vi "Confocal_0919.vi"() -> ()   [LabVIEW 2017]
uses:
  <vilib>/Math Plots/2D Math Plots/XY Plot Matrix/XY Plot Matrix XCtrl/XY Plot Matrix.xctl
  Public/Documents/SIToolkit/LabVIEW/ExamplesXX_4_3_1_4/Spectroscopy Applications/GlobalCamOpen.vi
  Public/Documents/SIToolkit/LabVIEW/ExamplesXX_4_3_1_4/Spectroscopy Applications/GlobalInitializeFlag.vi
  Program Files/SITK/SIToolkit/LabVIEW/ExamplesXX_4_3_1_4/Adv Applications/GlobalTimingMode.vi
  Public/Documents/SIToolkit/LabVIEW/ExamplesXX_4_3_1_4/Spectroscopy Applications/GlobalFramesToStr.vi
  Public/Documents/SIToolkit/LabVIEW/ExamplesXX_4_3_1_4/Spectroscopy Applications/GlobalAcquireFocusFlag.vi
  Public/Documents/SIToolkit/LabVIEW/ExamplesXX_4_3_1_4/Spectroscopy Applications/GlobalExposure.vi
  <vilib>/Math Plots/2D Math Plots/XY Plot Matrix/XY Plot Matrix Datatype/XY Plot Matrix Datatype.lvclass
panel:
  out "Position 7":dbl[](array[numeric]) format="%.6f"
  out "Position 4":dbl[](array[numeric]) format="%.6f"
  in  "error PI Stage":errorcluster
  out "error out 2":errorcluster
  in  "Tab Control":T1(tab)
  in  "Focus/Acquire Mode":u32=1 min=1 max=5 step=1
  in  "Number of Frames to store":u32=1 min=1 step=1
  in  "Timing Mode":u32(ring)=1 items=["N/A", "Free Run/Timed", "Trigger First (PM only)", "Ext Sync/Strobed ", "Variable Exp (PM only)", "Flash Mode (PM only)"]
  out "Pixel Time":i32
  out "Bit Depth":i32
  out "ReadOut port":i32
  out "ADC Speed":i32
  in  "Set Experiment \nParameters, Initialize \nCamera/Controller":bool
  out "Read Temp.":dbl format="%.2f"
  in  "Set Temp.":dbl format="%.2f"
  in  "Exposure 2":dbl=0.2 format="%.2f"
  out "Controller Initialized":bool
  in  "error in":errorcluster
  out "error out":errorcluster
  in  "Power":dbl=10.0
  in  "RF Power":bool=TRUE
  in  "Frequency":dbl=2810.0
  in  "Release Camera":bool
  out "Position 6":dbl[](array[numeric]) format="%.6f"
  out "Conn. Axis 5":string[](array[string])
  out "error out 3":errorcluster
  in  "stop":bool
  out "Read Frequency":dbl
  in  "Initial Frequency":dbl=2820.0
  in  "Final Frequency":dbl=2890.0
  in  "Step Size":dbl=3.0
  in  "OK Button 3":bool
  out "XY Plot Matrix":refnum<class "XY Plot Matrix Datatype.lvclass">[](xcontrol)
  out "history":dbl[][](array[numeric])
  in  "Number of Scans":i32
  in  "Serial Port":refnum<visa-resource-name>="COM3"
  out "COM Error":bool
  out "Camera Opened":bool
  out "Scan":i32
  in  "Number of Steps Left":dbl=5.0 format="%#_13g"
  in  "OK Button 5":bool
  in  "Step Size (microns)":dbl[](array[numeric])=[0.01]
  out "XY Plot Matrix":refnum<class "XY Plot Matrix Datatype.lvclass">[](xcontrol)
  in  "Number of Steps Down":dbl=5.0 format="%#_13g"
  out "Position":dbl[](array[numeric]) format="%.6f"
  out "Position 3":dbl[](array[numeric]) format="%.6f"
  in  "stop 2":bool
  out "Line Number":i32
  out "Position 2":dbl[](array[numeric]) format="%.6f"
  in  "?":bool
  out "Position 5":dbl[](array[numeric]) format="%.6f"
  in  "Step Size (microns) Y":dbl[](array[numeric])=[0.01]
  in  "Step Size (microns) X":dbl[](array[numeric])=[0.01]
  out "Position 8":dbl[](array[numeric]) format="%.6f"
  in  "?":bool
  in  "OK Button 4":bool
  in  "Frequency":dbl=2820.0
  out "XY Plot Matrix 2":refnum<class "XY Plot Matrix Datatype.lvclass">[](xcontrol) caption="XY Plot Matrix"
  out "history 2":dbl[][](array[numeric])
  in  "Points":i32=40
  in  "number of scans":i32=20
  out "Scan #":i32
  out "Point #":i32
  out "Acquire Graph":sgl[](graph)
  out "Collecting Data":bool
  in  "Full File Name for Acqure":path
  in  "OK Button":bool
  # "The following are read \nfrom camera after setting\nvalues to left.\n-1 value means item is not \nsupported by camera."
  # "Stage position on connection."
  # "Be sure to put in a full file name below before starting."
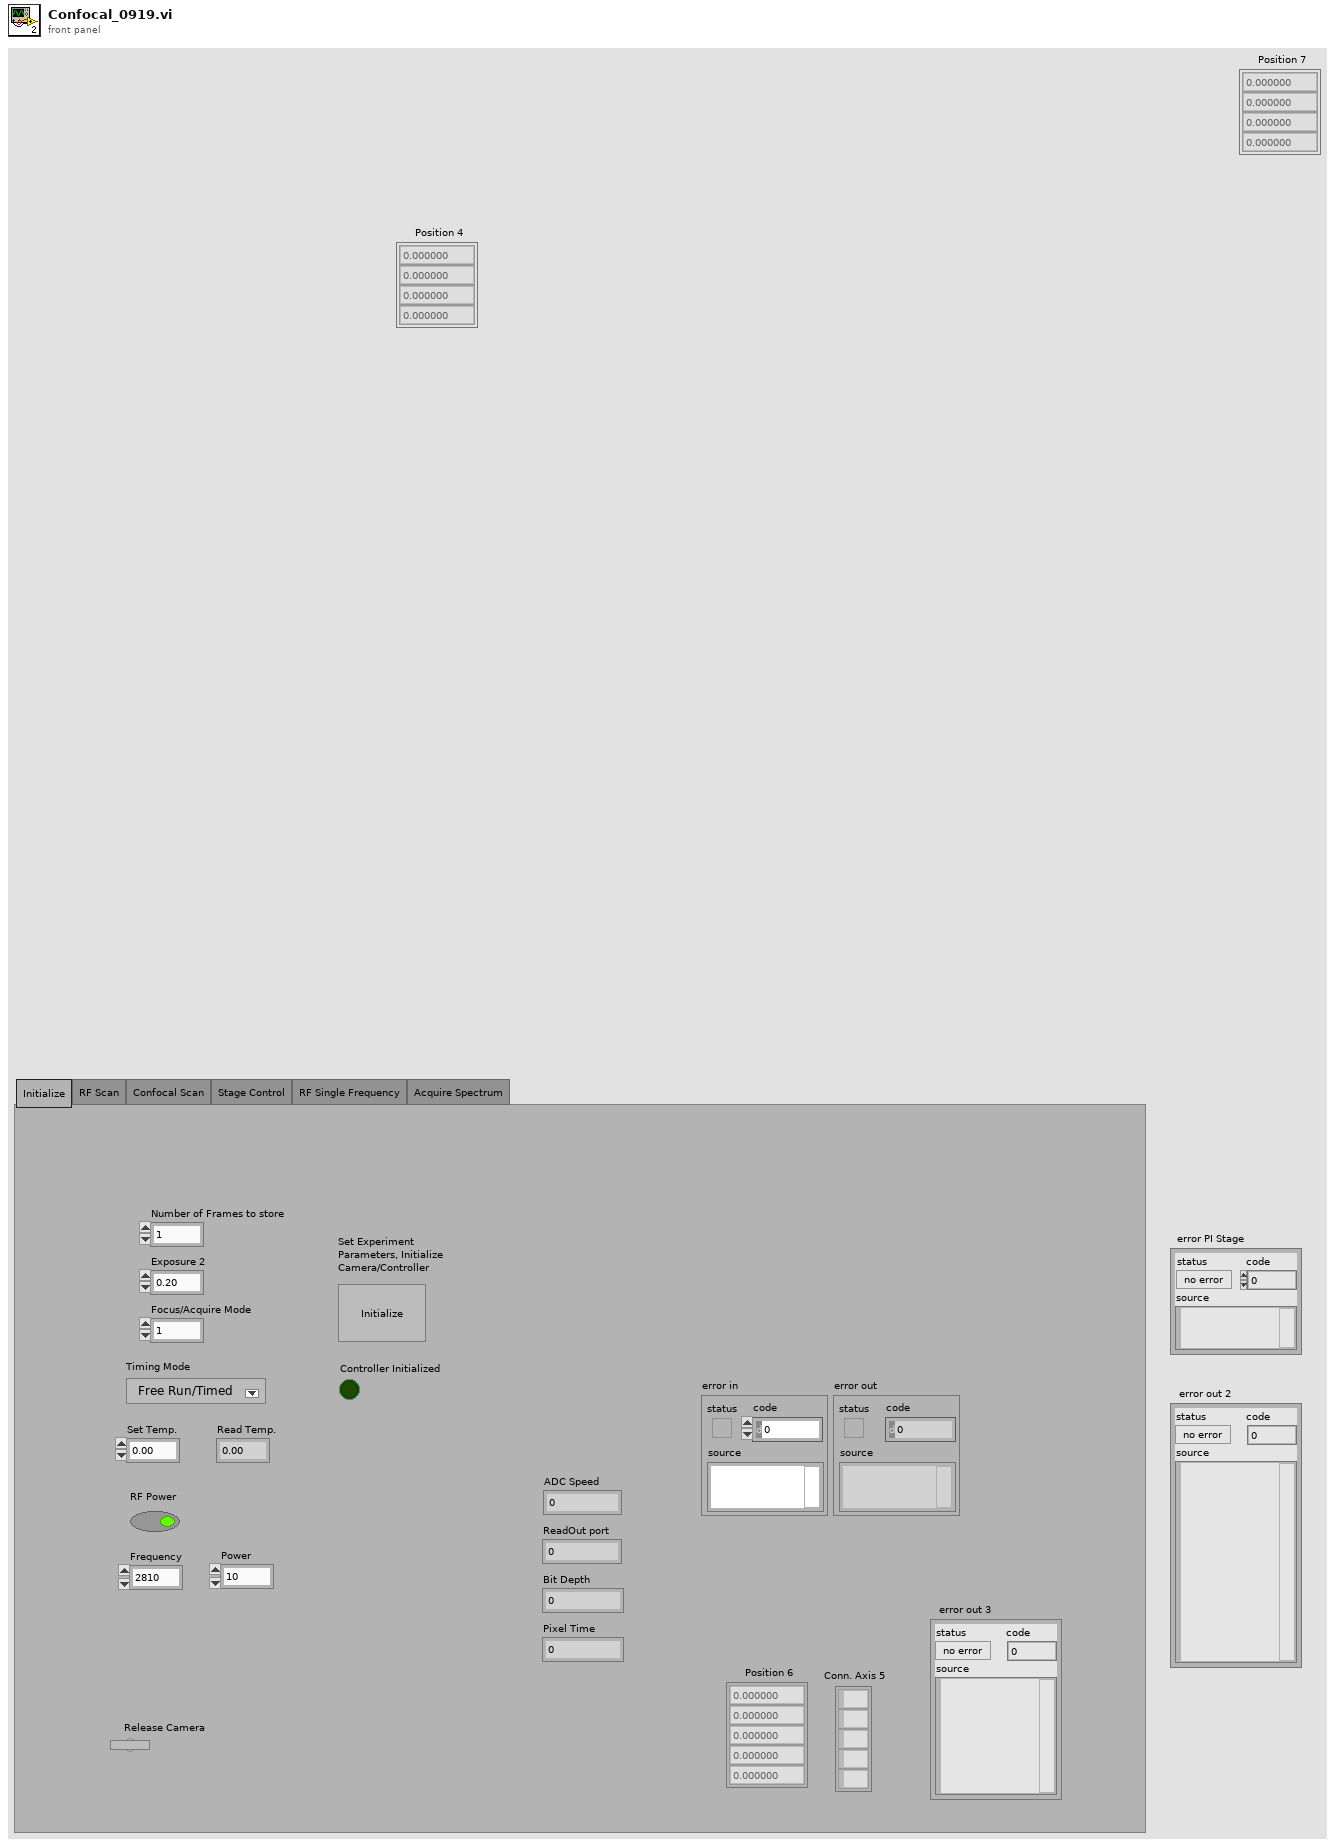
[diagram p1: front panel]
types:
  T1 = enum32{"Initialize", "RF Scan", "Confocal Scan", "Stage Control", "RF Single Frequency", "Acquire Spectrum"}
  T2 = cluster{"X start":u32, "X end":u32, "X Binning/Grouping":u32, "Y start":u32, "Y end":u32, "Y Binning/Grouping":u32}
  T3 = cluster{"Host address/name":string, "Port":i32, "Board":i32, "TCP/IP Search?":bool}
  T4 = cluster{"Camera Handle":u32, "Pulser Handle":u32, "File Handle":u32, "Display Handle":u32, "Image Handle":u32}
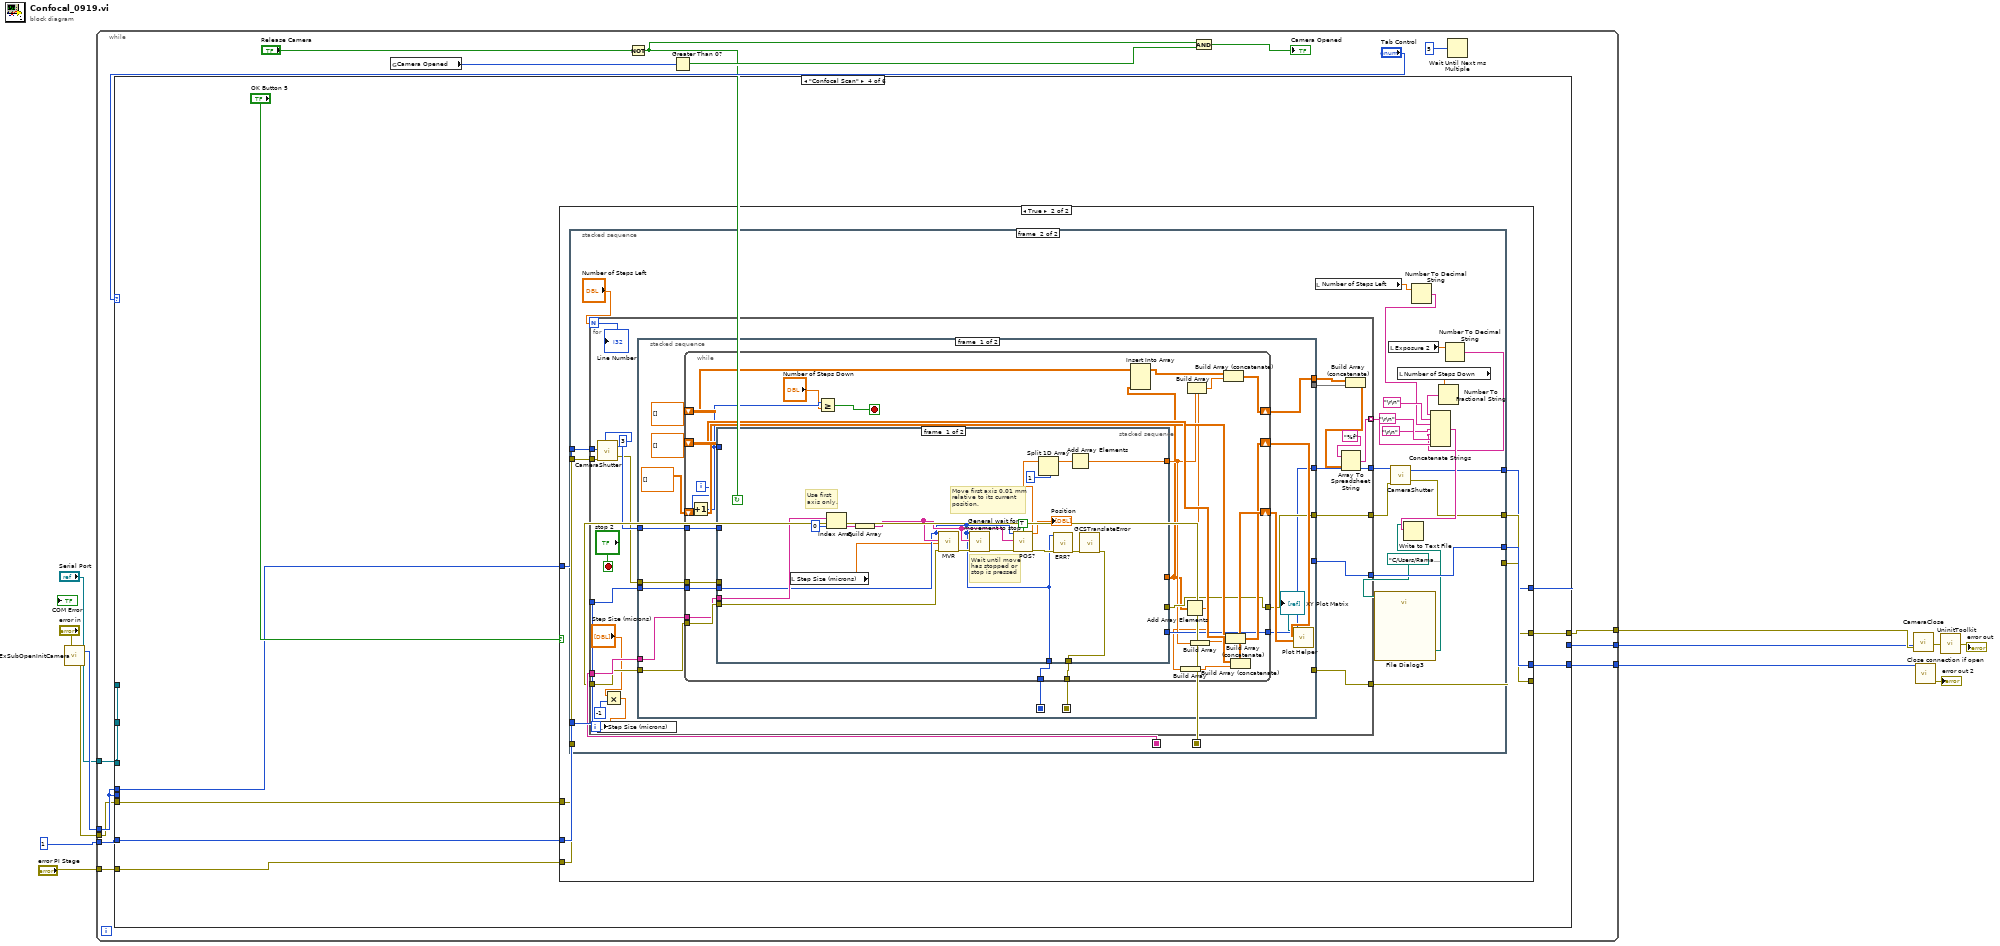
[diagram p0: block diagram]
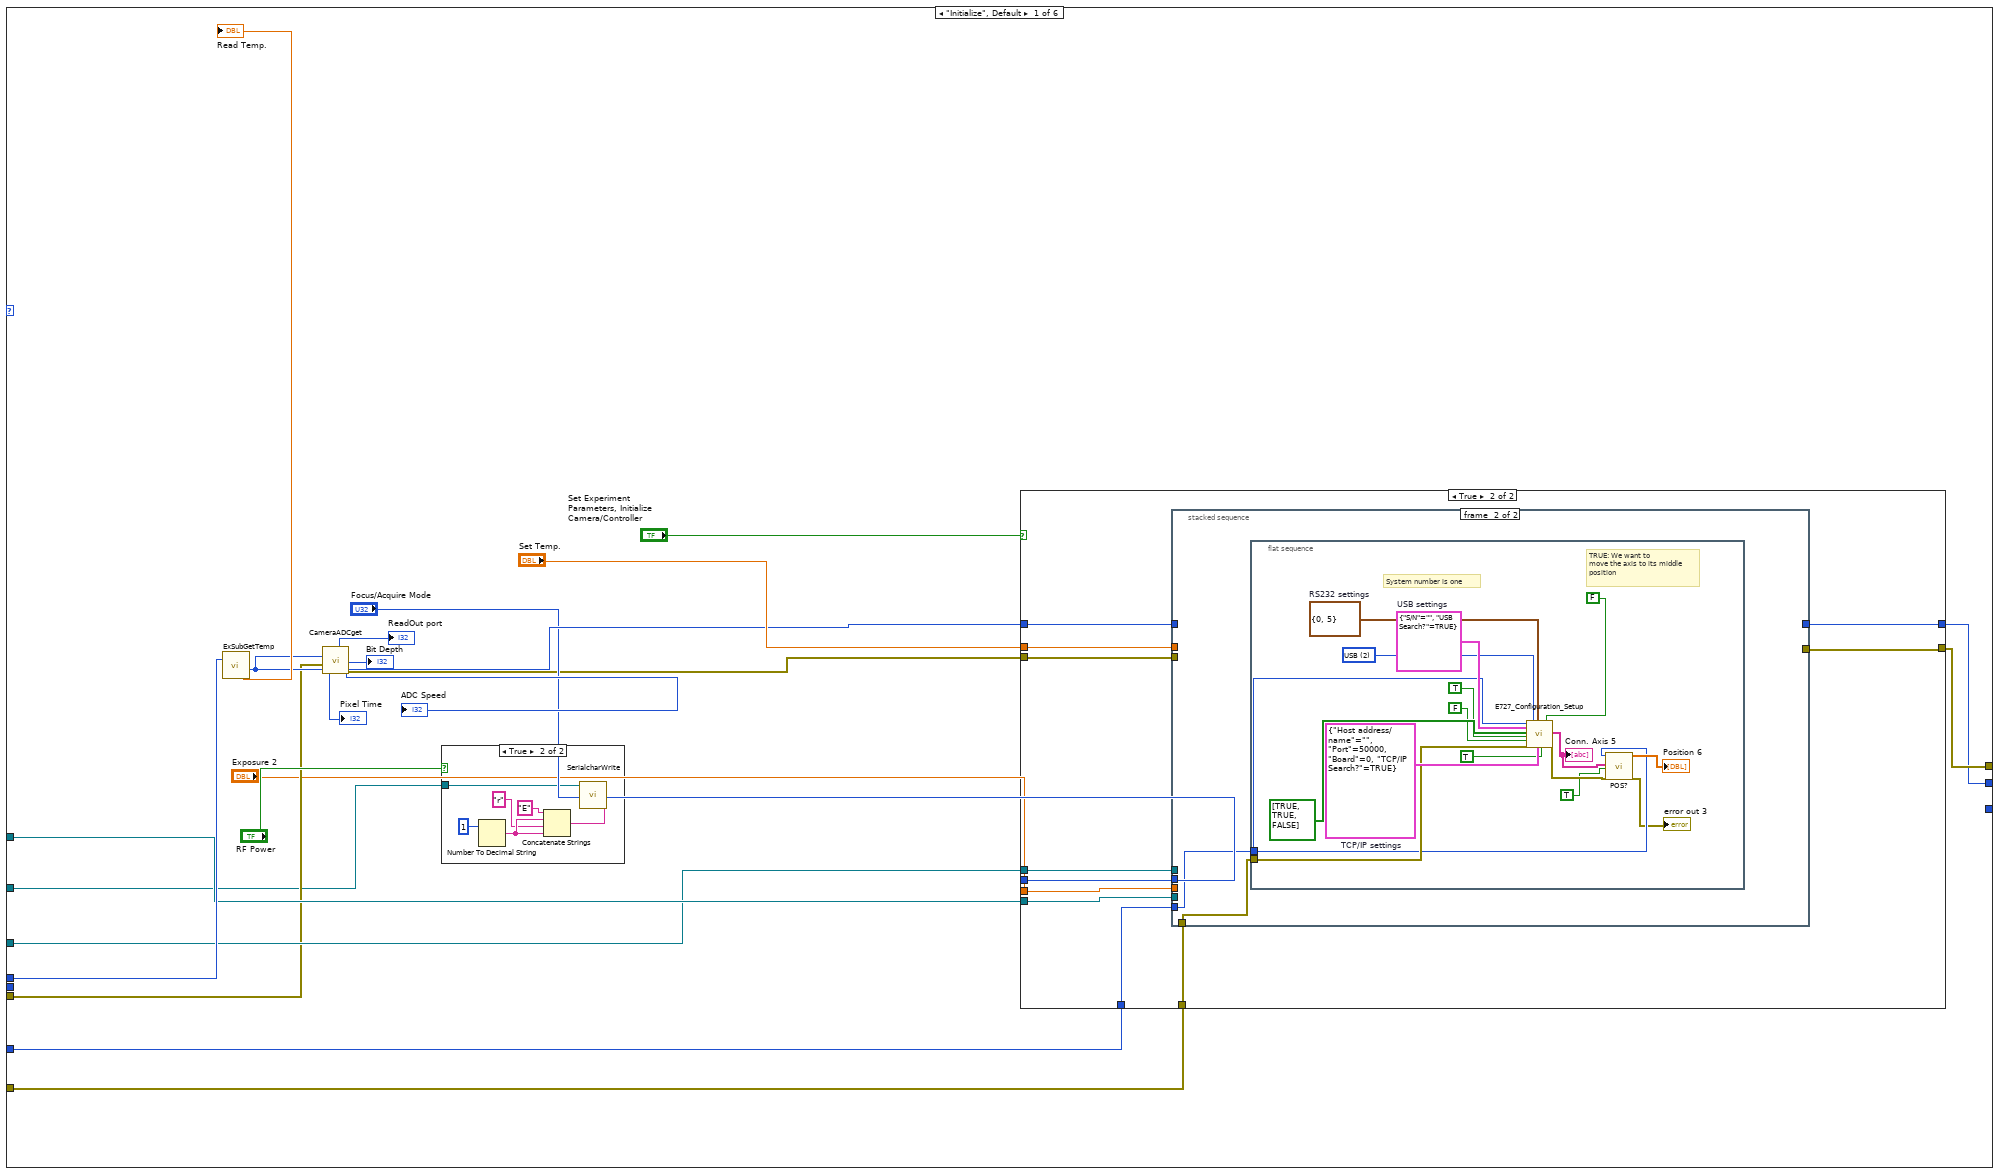
[diagram p2: hidden frame]
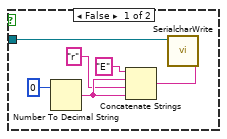
[diagram p3: hidden frame]
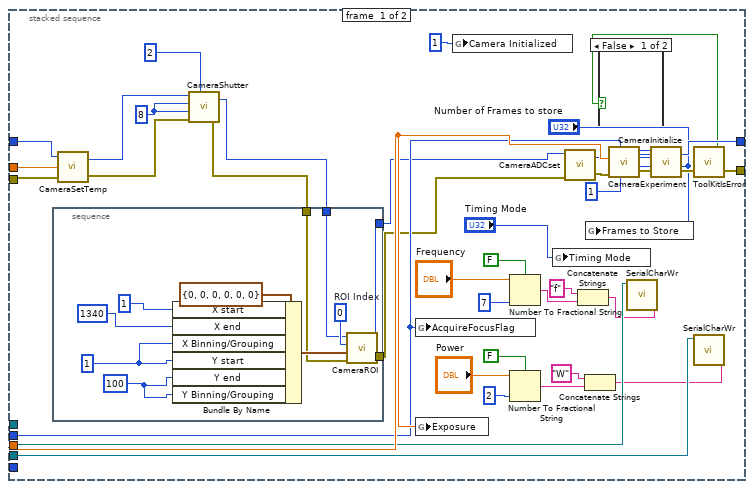
[diagram p5: hidden frame]
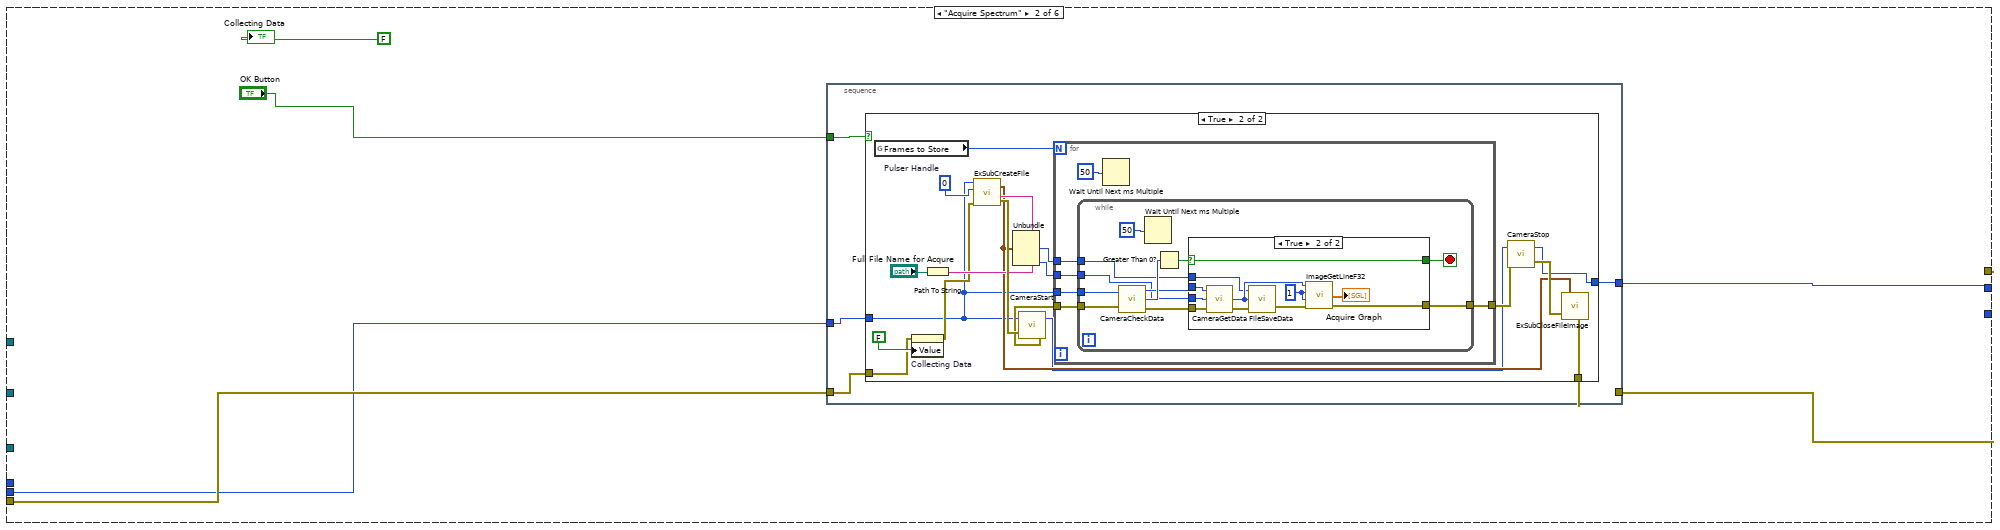
[diagram p7: hidden frame]
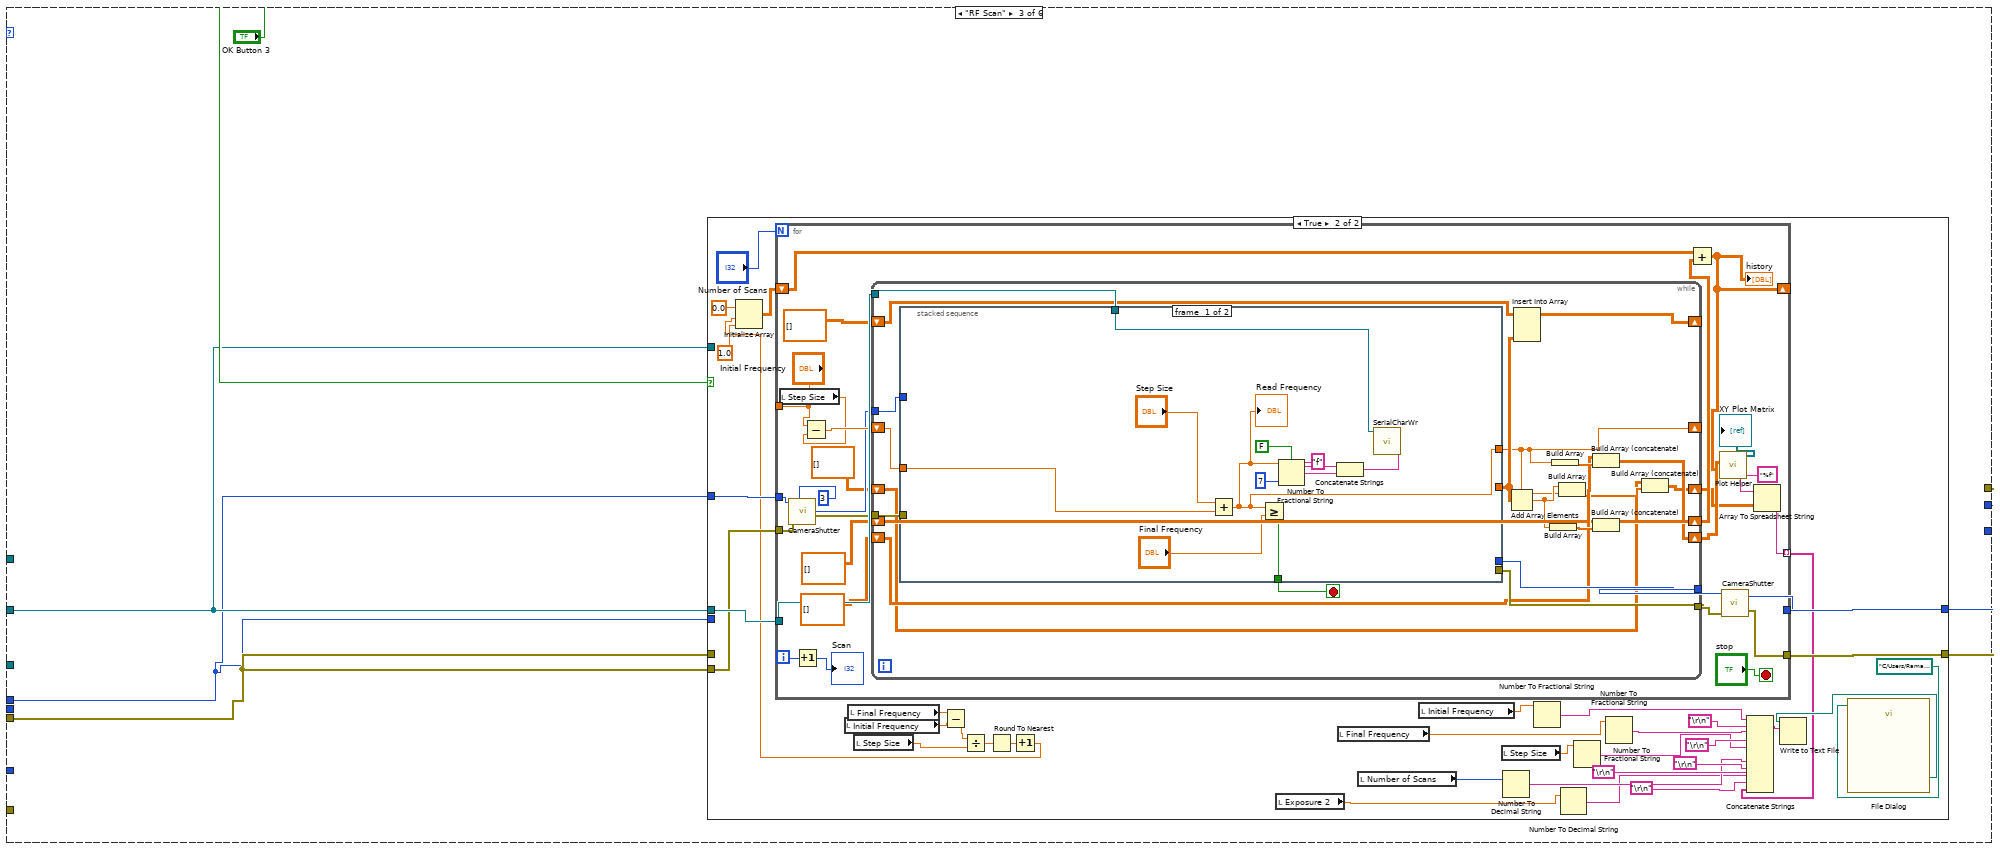
[diagram p10: hidden frame]
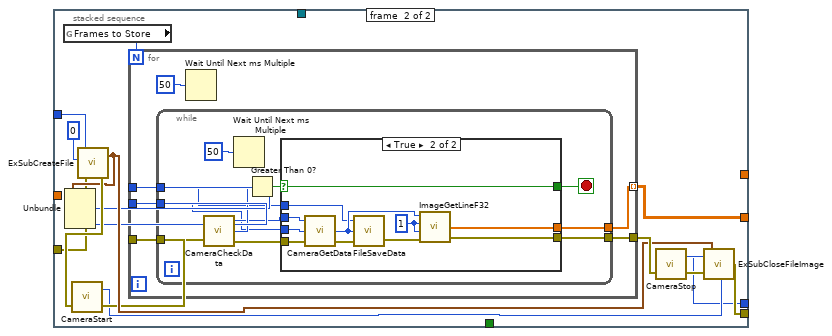
[diagram p12: hidden frame]
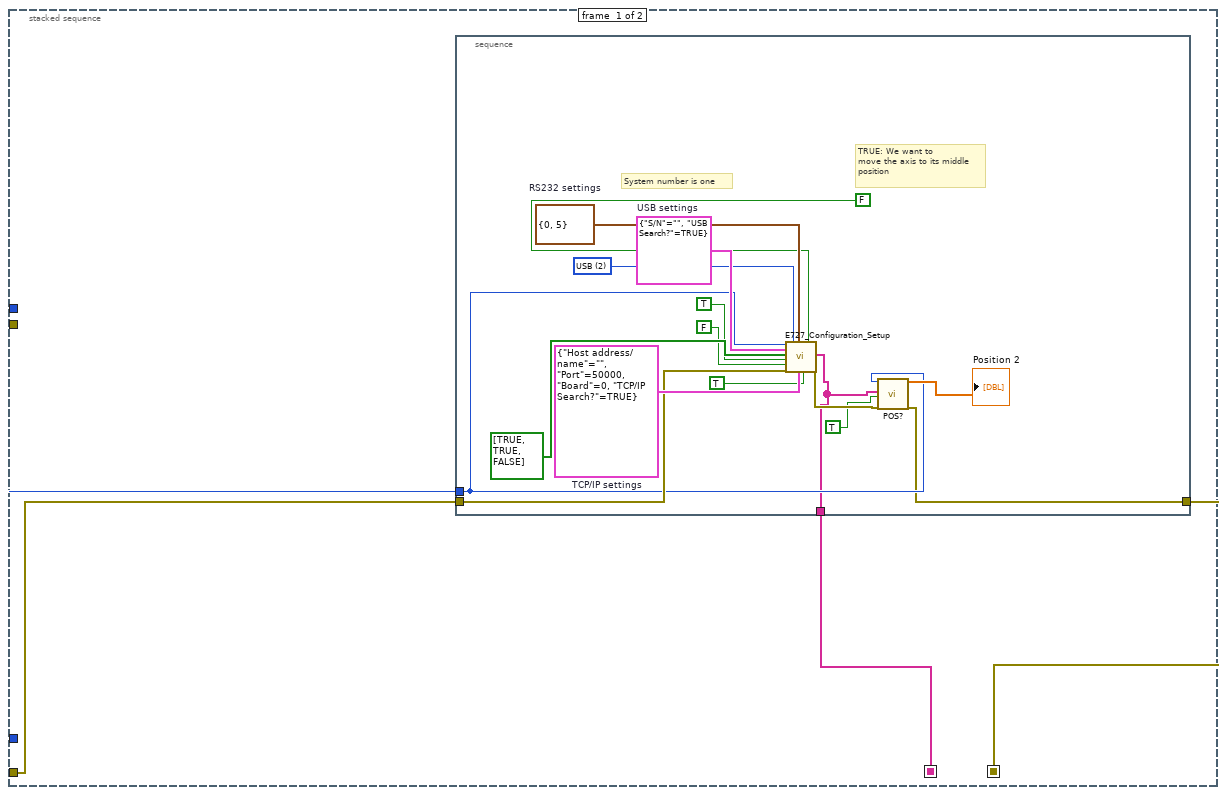
[diagram p15: hidden frame]
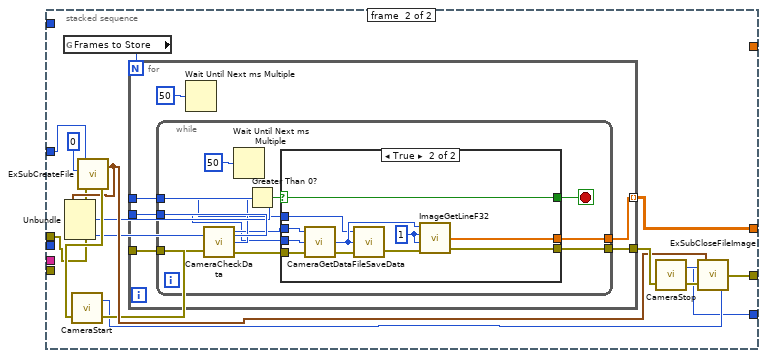
[diagram p16: hidden frame]
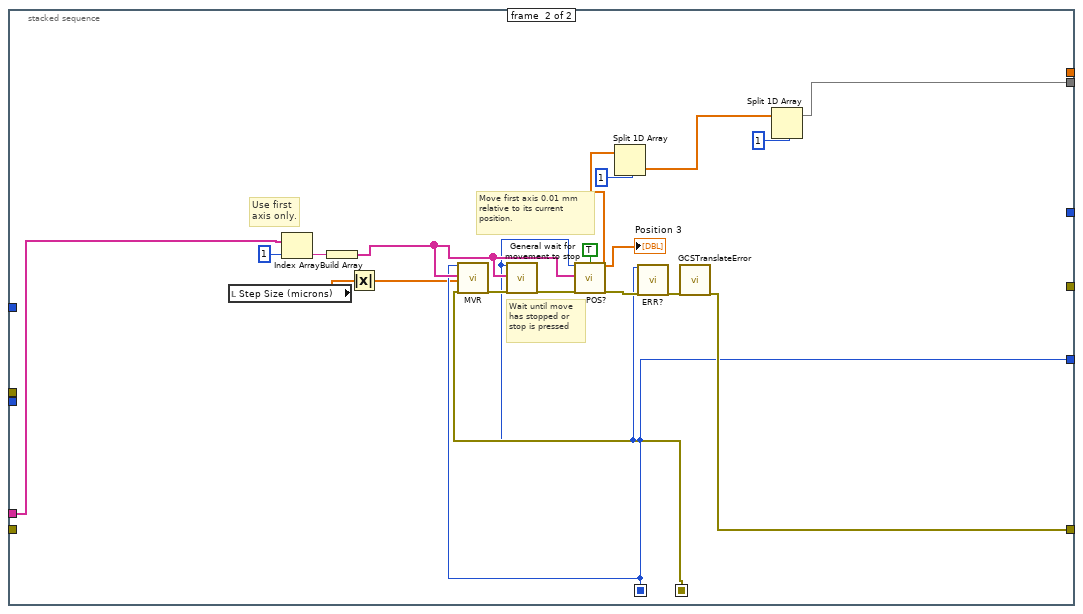
[diagram p18: hidden frame]
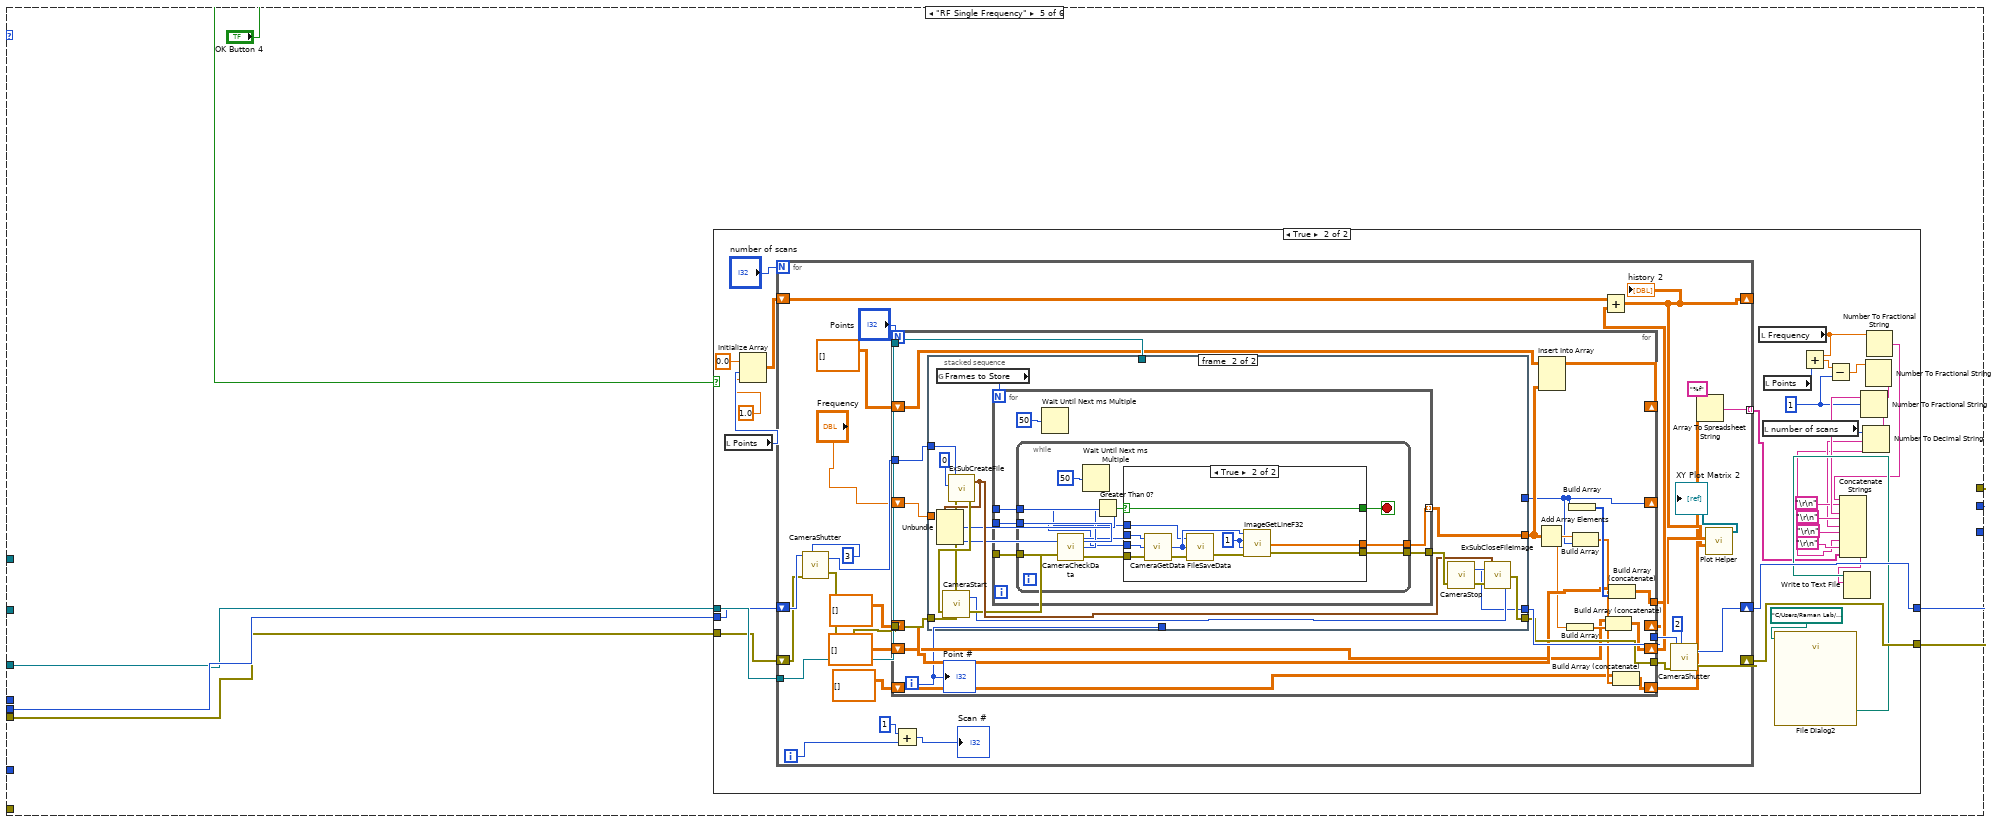
[diagram p19: hidden frame]
diagram:
  n1 = call "ExSubOpenInitCamera.vi"("error in (no error)"="error in") -> ("Camera Handle"=w11:u32, "error out"=w9:errorcluster)
  n2 = while {
    tunnel: w11 -> [w20]
    tunnel: "Serial Port" -> [w21]
    tunnel: w9 -> [w19]
    tunnel: [w18] -> w8
    tunnel: [w16] -> w5
    tunnel: "error PI Stage" -> [w15]
    tunnel: 1 -> [w13]
    tunnel: [w14] -> w1
    stop <- w17 continue-if-true
    n3 = case shown="\"Confocal Scan\"" "Tab Control" {
      tunnel: w20 -> [w40 _ w205 w353 _ _]
      tunnel: w21 -> [w34 _ w209 _ _ _]
      tunnel: w21 -> [w39 _ _ _ _ _]
      tunnel: w21 -> [w38 _ _ _ w562 _]
      tunnel: w20 -> [_ w147 _ _ w564 _]
      tunnel: w19 -> [w36 w148 w207 w354 w563 _]
      tunnel: [w30 w144 w206 w355 w561 _] -> w16
      tunnel: [w32 w145 w208 w356 w560 _] -> w18
      tunnel: w15 -> [w28 _ _ w358 _ w697]
      tunnel: w13 -> [w29 _ _ w360 _ w698]
      tunnel: [_ _ _ w359 _ _] -> w14
      frame "Initialize", Default {
        n4 = call "ExSubGetTemp.vi"("Camera Handle"=w40) -> ("Camera Handle"=w45:u32, "Temperature Real"=→"Read Temp.":dbl)  [unwired: 1 in, 1 out]
        n5 = call <userlib>:"CameraADCget.vi"("Camera handle"=w45, "error in (no error)"=w36) -> ("Bit Depth"=→"Bit Depth":i32, "Pixel Time"=→"Pixel Time":i32, "Readout Port"=→"ReadOut port":i32, "ADC Speed"=→"ADC Speed":i32, "error out"=w35:errorcluster)  [unwired: 3 out]
        n6 = case shown="True" "RF Power" {
          tunnel: w34 -> [w51 w58]
          frame False {
            n7 = Number To Decimal String(number=0) -> (decimal integer string=w56:string)  [unwired: 1 in]
            n8 = Concatenate Strings("E" ("element"), w56, "r" ("string"), w56) -> (w55:string)
            n9 = call "SerialcharWrite.vi"("VISA resource name"=w51, "write buffer"=w55) -> ()  [unwired: 8 in, 1 out]
          }
          frame True {
            n10 = Number To Decimal String(number=1) -> (decimal integer string=w60:string)  [unwired: 1 in]
            n11 = Concatenate Strings("E" ("element"), w60, "r" ("string"), w60) -> (w61:string)
            n12 = call "SerialcharWrite.vi"("VISA resource name"=w58, "write buffer"=w61) -> ()  [unwired: 8 in, 1 out]
          }
        }
        n13 = case shown="True" "Set Experiment \nParameters, Initialize \nCamera/Controller" {
          tunnel: "Exposure 2" -> [_ w73]
          tunnel: "Set Temp." -> [_ w74]
          tunnel: w45 -> [w64 w75]
          tunnel: [w64 w72] -> w30
          tunnel: "Focus/Acquire Mode" -> [_ w71]
          tunnel: w39 -> [_ w70]
          tunnel: w38 -> [_ w69]
          tunnel: w35 -> [w63 w68]
          tunnel: [w63 w67] -> w32
          tunnel: w29 -> [_ w66]
          tunnel: w28 -> [_ w65]
          frame False {
          }
          frame True {
            n14 = stacked-sequence {
              tunnel: w75 -> [w114 _]
              tunnel: w74 -> [w113 _]
              tunnel: w73 -> [w112 _]
              tunnel: [w111 _] -> w72
              tunnel: w71 -> [w110 _]
              tunnel: w70 -> [w109 _]
              tunnel: w69 -> [w108 _]
              tunnel: w68 -> [w107 _]
              tunnel: [w106 _] -> w67
              tunnel: w66 -> [_ w126]
              tunnel: w65 -> [_ w127]
              frame #0 {
                w76 = 8
                n15 = call <userlib>:"CameraSetTemp.vi"("error in (no error)"=w107, "Temperature"=w113, "Camera Handle"=w114) -> ("error out"=w79:errorcluster, "Camera Handle"=w81:u32)
                n16 = call <userlib>:"CameraShutter.vi"("Camera Handle"=w81, "Shutter Comp Time: Pre Open"=w76, "Shutter Comp Time: Post Open"=w76, "error in"=w79, "Shutter State"=2) -> ("Camera Handle"=w80:u32, "error out"=w78:errorcluster)
                n17 = stacked-sequence {
                  tunnel: [w122] -> w83
                  tunnel: w80 -> [w119]
                  tunnel: w78 -> [w118]
                  tunnel: [w117] -> w82
                  frame #0 {
                    w121 = 100
                    w115 = 1
                    w124 = u32 0  # ROI Index
                    n18 = Bundle By Name(cluster=T2 {"X start"=0, "X end"=0, "X Binning/Grouping"=0, "Y start"=0, "Y end"=0, "Y Binning/Grouping"=0} ("ROI Params"), "X start"=1, "X end"=1340, "X Binning/Grouping"=w115, "Y start"=w115, "Y end"=w121, "Y Binning/Grouping"=w121) -> (w125:T2)
                    n19 = call <userlib>:"CameraROI.vi"("error in"=w118, "ROI Params"=w125, "ROI Index"=w124, "Camera Handle"=w119) -> ("error out"=w117:errorcluster, "Camera Handle"=w122:u32)
                  }
                }
                n20 = global write "GlobalAcquireFocusFlag.vi" "AcquireFocusFlag"(w110) -> ()
                n21 = global write "GlobalExposure.vi" "Exposure"(w112) -> ()
                n22 = global write "GlobalInitializeFlag.vi" "Camera Initialized"(1) -> ()
                n23 = Number To Fractional String(use system decimal point (T)=FALSE, number="Frequency", precision (6)=7) -> (F-format string=w85:string)  [unwired: 1 in]
                n24 = Number To Fractional String(use system decimal point (T)=FALSE, number="Power", precision (6)=2) -> (F-format string=w93:string)  [unwired: 1 in]
                n25 = global write "GlobalTimingMode.vi" "Timing Mode"("Timing Mode") -> ()
                n26 = call <userlib>:"CameraADCset.vi"("error in (no error)"=w82, "Camera Handle"=w83) -> ("error out"=w102:errorcluster, "Camera Handle"=w101:u32)  [unwired: 4 in]
                n27 = Concatenate Strings("f", w85) -> (w91:string)
                n28 = Concatenate Strings("W", w93) -> (w94:string)
                n29 = global write "GlobalFramesToStr.vi" "Frames to Store"("Number of Frames to store") -> ()
                n30 = call <userlib>:"CameraExperiment.vi"("Number of Accumulations"=1, "Acquire / Focus Flag"=w110, "error in"=w102, "Number of Images"="Number of Frames to store", "Exposure (sec)"=w112, "Camera Handle"=w101) -> ("error out"=w100:errorcluster, "Camera Handle"=w99:u32)
                n31 = call "SerialCharWr.vi"("VISA resource name"=w108, "write buffer"=w91) -> ()  [unwired: 6 in, 3 out]
                n32 = call <userlib>:"CameraInitialize.vi"("error in"=w100, "Camera Handle"=w99) -> ("error out"=w97:errorcluster, "Camera Handle"=w111:u32)
                n33 = call <userlib>:"ToolKitIsError.vi"("error in"=w97) -> ("error out"=w106:errorcluster, "Error Flag"=w98:bool)  [unwired: 1 in]
                n34 = case shown="False" w98 {
                  frame False {
                  }
                  frame True {
                  }
                }
                n35 = call "SerialCharWr.vi"("VISA resource name"=w109, "write buffer"=w94) -> ()  [unwired: 6 in, 3 out]
              }
              frame #1 {
                n36 = flat-sequence {
                  tunnel: w127 -> [w131]
                  tunnel: w126 -> [w130]
                  frame #0 {
                    w143 = cluster{"S/N":string, "USB Search?":bool} {"S/N"="", "USB Search?"=TRUE}  # USB settings
                    w139 = u16 2 items=["RS232", "TCP/IP", "USB"] ("Interface")
                    w138 = cluster{"Portnumber":i32, "Baudrate":u16} {"Portnumber"=0, "Baudrate"=5}  # RS232 settings
                    w137 = T3 {"Host address/name"="", "Port"=50000, "Board"=0, "TCP/IP Search?"=TRUE}  # TCP/IP settings
                    # "TRUE: We want to\nmove the axis to its middle\nposition"
                    # "System number is one"
                    n37 = call "E727_Configuration_Setup.vi"("System no."=w130, "USB settings"=w143, "Are stages connected?"=bool[] [TRUE, TRUE, FALSE], "Change servo status to ON?"=TRUE ("Use dialog to define\nconnected stages?"), "Perform autozero?"=FALSE ("Use dialog to define\nconnected stages?"), "error in"=w131, "Interface"=w139, "RS232 settings"=w138, "TCP/IP settings"=w137, "Stop wave generator\noutput (if any)"=TRUE ("All axes?"), "Move to middle?"=FALSE) -> ("All conn. axes"=w129:string[], "error out"=w133:errorcluster)  [unwired: 3 in, 4 out]
                    "Conn. Axis 5" <- w129
                    n38 = call "POS?.vi"("System no."=w130, "Axes to query"=w129, "All axes?"=TRUE, "error in"=w133) -> ("Position"=→"Position 6":dbl[], "error out"=→"error out 3":errorcluster)  [unwired: 1 in, 13 out]
                  }
                }
              }
            }
          }
        }
        n39 = global read "GlobalInitializeFlag.vi" "Camera Initialized"() -> (w48:u32)
        n40 = Greater Than 0?(x=w48) -> (x > 0?=→"Controller Initialized":bool)
      }
      frame "Acquire Spectrum" {
        n41 = stacked-sequence {
          tunnel: [w151] -> w145
          tunnel: [w152] -> w144
          tunnel: w148 -> [w154]
          tunnel: "OK Button" -> [w153]
          tunnel: w147 -> [w150]
          frame #0 {
            n42 = case shown="True" w153 {
              tunnel: [w155 w167] -> w152
              tunnel: [w156 w159] -> w151
              tunnel: w154 -> [w156 w158]
              tunnel: w150 -> [w155 w157]
              frame False {
              }
              frame True {
                w161 = u32 0  # Pulser Handle
                n43 = global read "GlobalFramesToStr.vi" "Frames to Store"() -> (w170:u32)
                n44 = property on="Collecting Data" class="Bool (strict)"(error in=w158, "Value"=FALSE) -> (error out=w169:errorcluster)  [unwired: 1 in, 1 out]
                n45 = Path To String(path="Full File Name for Acqure") -> (string=w172:string)
                n46 = call "ExSubCreateFile.vi"("error in (no error)"=w169, "File and Display Name"=w172, "Pulser Handle"=w161, "Camera Handle"=w157) -> ("error out"=w174:errorcluster, "Handles Out"=w165:T4)
                n47 = Unbundle(w165) -> ("File Handle"=w160:u32, "Image Handle"=w163:u32)  [unwired: 3 out]
                n48 = call <userlib>:"CameraStart.vi"("error in"=w174, "Camera Handle"=w157) -> ("error out"=w164:errorcluster, "Camera Handle"=w162:u32)
                n49 = for {
                  N: w170 -> [_]
                  tunnel: w157 -> [w179]
                  tunnel: w164 -> [w178]
                  tunnel: [w177] -> w166
                  tunnel: w160 -> [w176]
                  tunnel: w163 -> [w175]
                  n50 = while {
                    tunnel: [w186] -> w177
                    tunnel: w179 -> [w184]
                    tunnel: w178 -> [w183]
                    tunnel: w176 -> [w182]
                    tunnel: w175 -> [w181]
                    stop <- w187 stop-if-true
                    n51 = call <userlib>:"CameraCheckData.vi"("Camera Handle"=w184, "error in"=w183) -> ("Camera Handle"=w189:u32, "Number Of Frames Available"=w191:i32, "error out"=w188:errorcluster)
                    n52 = Wait Until Next ms Multiple(millisecond multiple=u32 50) -> ()  [unwired: 1 out]
                    n53 = Greater Than 0?(x=w191) -> (x > 0?=w190:bool)
                    n54 = case shown="True" w190 {
                      selector: w190 -> [w192 w202]
                      tunnel: w189 -> [_ w204]
                      tunnel: w188 -> [w193 w203]
                      tunnel: [w192 w202] -> w187
                      tunnel: [w193 w197] -> w186
                      tunnel: w182 -> [_ w195]
                      tunnel: w181 -> [_ w194]
                      frame False {
                      }
                      frame True {
                        w198 = 1
                        n55 = call <userlib>:"CameraGetData.vi"("error in"=w203, "Image/Data Handle"=w194, "Camera Handle"=w204) -> ("error out"=w201:errorcluster, "Image/Data Handle"=w199:u32)  [unwired: 1 out]
                        n56 = call <userlib>:"FileSaveData.vi"("error in"=w201, "Image Handle"=w199, "File Handle"=w195) -> ("error out"=w200:errorcluster)  [unwired: 1 out]
                        n57 = call <userlib>:"ImageGetLineF32.vi"("error in"=w200, "Z Position"=w198, "Y Position"=w198, "Data Handle"=w199) -> ("error out"=w197:errorcluster, "Array F32"=→"Acquire Graph":sgl[])  [unwired: 1 out]
                      }
                    }
                  }
                  n58 = Wait Until Next ms Multiple(millisecond multiple=u32 50) -> ()  [unwired: 1 out]
                }
                n59 = call <userlib>:"CameraStop.vi"("error in"=w166, "Camera Handle"=w162) -> ("error out"=w171:errorcluster, "Camera Handle"=w167:u32)
                n60 = call "ExSubCloseFileImage.vi"("error in (no error)"=w171, "Handles In"=w165) -> ("error out"=w159:errorcluster)
              }
            }
          }
        }
        "Collecting Data" <- FALSE
      }
      frame "RF Scan" {
        n61 = case shown="True" "OK Button 3" {
          tunnel: w209 -> [_ _]
          tunnel: w205 -> [w212 _]
          tunnel: w207 -> [w211 _]
          tunnel: w209 -> [_ w247]
          tunnel: [w212 w232] -> w206
          tunnel: [w211 w231] -> w208
          tunnel: w205 -> [_ w234]
          tunnel: w207 -> [_ w233]
          frame False {
          }
          frame True {
            n62 = local read "Initial Frequency"() -> (w222:dbl)
            n63 = local read "Final Frequency"() -> (w223:dbl)
            n64 = local read "Step Size"() -> (w220:dbl)
            n65 = Subtract(x=w223, y=w222) -> (x-y=w221:dbl)
            n66 = Divide(x=w221, y=w220) -> (x/y=w219:dbl)
            n67 = Round To Nearest(number=w219) -> (nearest integer value=w218:dbl)
            n68 = Increment(x=w218) -> (x+1=w217:dbl)
            n69 = Initialize Array(0.0, w217, 1.0) -> (w225:dbl[][])
            n70 = for {
              N: "Number of Scans" -> [_]
              tunnel: w247 -> [w275]
              tunnel: w234 -> [w268]
              tunnel: w233 -> [w267]
              tunnel: [w263] -> w232
              tunnel: [w262] -> w231
              shift-right: [w253] -> _
              shift-left: w225 -> [w257]
              tunnel: ["Initial Frequency"] -> _
              tunnel: [w252] -> w216 mode=indexing
              i -> [w259]
              stop <- "stop" stop-if-true
              n71 = local read "Step Size"() -> (w269:dbl)
              n72 = call <userlib>:"CameraShutter.vi"("Camera Handle"=w268, "error in"=w267, "Shutter State"=3) -> ("Camera Handle"=w264:u32, "error out"=w265:errorcluster)  [unwired: 2 in]
              n73 = Increment(x=w259) -> (x+1=→"Scan":i32)
              n74 = Subtract(x="Initial Frequency", y=w269) -> (x-y=w274:dbl)
              n75 = while {
                shift-right: [w280] -> _
                shift-left: w274 -> [w293]
                tunnel: w275 -> [w296]
                tunnel: [w295] -> w271
                tunnel: [w294] -> w270
                shift-right: [w289] -> _
                shift-left: dbl[][] [] -> [w290]
                tunnel: w265 -> [w292]
                tunnel: w264 -> [w291]
                shift-right: [w282] -> w255
                shift-left: dbl[][] [] -> [w286]
                shift-right: [w283] -> w256
                shift-left: dbl[][] [] -> [w284]
                shift-right: [w277] -> w249
                shift-left: dbl[][] [] -> [w278]
                stop <- w276 stop-if-true
                n76 = stacked-sequence {
                  tunnel: w296 -> [w301 _]
                  tunnel: w293 -> [w300 _]
                  tunnel: [_ w311] -> w295
                  tunnel: [_ w312] -> w294
                  tunnel: [w299 _] -> w280
                  tunnel: [_ w310] -> w285
                  tunnel: w292 -> [_ w309]
                  tunnel: w291 -> [_ w308]
                  tunnel: [w297 _] -> w276
                  frame #0 {
                    n77 = Add(x="Step Size", y=w300) -> (x+y=w299:dbl)
                    "Read Frequency" <- w299
                    n78 = Greater Or Equal?(x=w299, y="Final Frequency") -> (x >= y?=w297:bool)
                    n79 = Number To Fractional String(use system decimal point (T)=FALSE, number=w299, precision (6)=7) -> (F-format string=w306:string)  [unwired: 1 in]
                    n80 = Concatenate Strings("f", w306) -> (w307:string)
                    n81 = call "SerialCharWr.vi"("VISA resource name"=w301, "write buffer"=w307) -> ()  [unwired: 6 in, 3 out]
                  }
                  frame #1 {
                    n82 = global read "GlobalFramesToStr.vi" "Frames to Store"() -> (w320:u32)
                    n83 = call "ExSubCreateFile.vi"("error in (no error)"=w309, "Pulser Handle"=u32 0, "Camera Handle"=w308) -> ("error out"=w322:errorcluster, "Handles Out"=w318:T4)  [unwired: 1 in]
                    n84 = Unbundle(w318) -> ("File Handle"=w313:u32, "Image Handle"=w316:u32)  [unwired: 3 out]
                    n85 = call <userlib>:"CameraStart.vi"("error in"=w322) -> ("error out"=w317:errorcluster, "Camera Handle"=w315:u32)  [unwired: 1 in]
                    n86 = for {
                      N: w320 -> [_]
                      tunnel: w317 -> [w327]
                      tunnel: [w326] -> w319
                      tunnel: w313 -> [w325]
                      tunnel: w316 -> [w324]
                      tunnel: [w323] -> w310 mode=indexing
                      n87 = while {
                        tunnel: [w334] -> w326
                        tunnel: w327 -> [w332]
                        tunnel: w325 -> [w331]
                        tunnel: w324 -> [w330]
                        tunnel: [w329] -> w323
                        stop <- w335 stop-if-true
                        n88 = call <userlib>:"CameraCheckData.vi"("error in"=w332) -> ("Camera Handle"=w337:u32, "Number Of Frames Available"=w339:i32, "error out"=w336:errorcluster)  [unwired: 1 in]
                        n89 = Wait Until Next ms Multiple(millisecond multiple=u32 50) -> ()  [unwired: 1 out]
                        n90 = Greater Than 0?(x=w339) -> (x > 0?=w338:bool)
                        n91 = case shown="True" w338 {
                          selector: w338 -> [w340 w350]
                          tunnel: w337 -> [_ w352]
                          tunnel: w336 -> [w341 w351]
                          tunnel: [w340 w350] -> w335
                          tunnel: [w341 w345] -> w334
                          tunnel: w331 -> [_ w344]
                          tunnel: w330 -> [_ w343]
                          tunnel: [_ w342] -> w329
                          frame False {
                          }
                          frame True {
                            w346 = 1
                            n92 = call <userlib>:"CameraGetData.vi"("error in"=w351, "Image/Data Handle"=w343, "Camera Handle"=w352) -> ("error out"=w349:errorcluster, "Image/Data Handle"=w347:u32)  [unwired: 1 out]
                            n93 = call <userlib>:"FileSaveData.vi"("error in"=w349, "Image Handle"=w347, "File Handle"=w344) -> ("error out"=w348:errorcluster)  [unwired: 1 out]
                            n94 = call <userlib>:"ImageGetLineF32.vi"("error in"=w348, "Z Position"=w346, "Y Position"=w346, "Data Handle"=w347) -> ("error out"=w345:errorcluster, "Array F32"=w342:sgl[])  [unwired: 1 out]
                          }
                        }
                      }
                      n95 = Wait Until Next ms Multiple(millisecond multiple=u32 50) -> ()  [unwired: 1 out]
                    }
                    n96 = call <userlib>:"CameraStop.vi"("error in"=w319, "Camera Handle"=w315) -> ("error out"=w321:errorcluster, "Camera Handle"=w311:u32)
                    n97 = call "ExSubCloseFileImage.vi"("error in (no error)"=w321, "Handles In"=w318) -> ("error out"=w312:errorcluster)
                  }
                }
                n98 = Add Array Elements(numeric array=w285) -> (sum=w281:sgl)
                n99 = Insert Into Array(array=w290, new element=w285) -> (w289:dbl[][])  [unwired: 2 in]
                n100 = Build Array(w281) -> (w287:sgl[])
                n101 = Build Array(w280) -> (w288:dbl[])
                n102 = Build Array(w281, w280) -> (w279:dbl[])
                n103 = Build Array (concatenate)(w286, w288) -> (w282:dbl[][])
                n104 = Build Array (concatenate)(w284, w287) -> (w283:dbl[][])
                n105 = Build Array (concatenate)(w278, w279) -> (w277:dbl[][])
              }
              n106 = Add(x=w257, y=w256) -> (x+y=w253:dbl[][])
              "history" <- w253
              n107 = call <vilib>:"Plot Helper.vi"("y matrix"=w253, "x matrix"=w255) -> ("2D Plotmatrix Class Obj Array out"=→"XY Plot Matrix":refnum<class "XY Plot Matrix Datatype.lvclass">[])  [unwired: 2 in, 7 out]
              n108 = call <userlib>:"CameraShutter.vi"("Camera Handle"=w271, "error in"=w270) -> ("Camera Handle"=w263:u32, "error out"=w262:errorcluster)  [unwired: 3 in]
              n109 = Array To Spreadsheet String(array=w249, 3:"%f" ("format string")) -> (spreadsheet string=w252:string)  [unwired: 1 in]
            }
            n110 = local read "Exposure 2"() -> (w213:dbl)
            n111 = local read "Final Frequency"() -> (w229:dbl)
            n112 = local read "Number of Scans"() -> (w227:i32)
            n113 = local read "Initial Frequency"() -> (w228:dbl)
            n114 = local read "Step Size"() -> (w230:dbl)
            n115 = Number To Decimal String(number=w227) -> (decimal integer string=w235:string)  [unwired: 1 in]
            n116 = Number To Fractional String(number=w228) -> (F-format string=w245:string)  [unwired: 3 in]
            n117 = Number To Decimal String(number=w213) -> (decimal integer string=w214:string)  [unwired: 1 in]
            n118 = Number To Fractional String(number=w230) -> (F-format string=w240:string)  [unwired: 3 in]
            n119 = Number To Fractional String(number=w229) -> (F-format string=w239:string)  [unwired: 3 in]
            n120 = Concatenate Strings(w245, "\r\n", w239, "\r\n", w240, "\r\n", w235, "\r\n", w214, "\r\n", w216) -> (w243:string)
            n121 = call "File Dialog"("start path"=path "C:/Users/Raman Lab/Desktop/Molly") -> ("selected path"=w238:path)  [unwired: 11 in, 3 out]
            n122 = Write to Text File(file (use dialog)=w238, text=w243) -> ()  [unwired: 2 in, 3 out]
          }
        }
      }
      frame "Confocal Scan" {
        n123 = case shown="True" "OK Button 5" {
          tunnel: w360 -> [_ w368]
          tunnel: [_ w367] -> w359
          tunnel: [_ w366] -> _
          tunnel: w358 -> [_ w365]
          tunnel: [_ w364] -> w356
          tunnel: [_ w363] -> w355
          tunnel: w354 -> [_ w362]
          tunnel: w353 -> [_ w361]
          frame False {
          }
          frame True {
            n124 = stacked-sequence {
              seq-local: [w370 _] -> [_ w410]
              seq-local: [w369 _] -> [_ w409]
              tunnel: w368 -> [w371 w413]
              tunnel: [_ w412] -> w367
              tunnel: [_ w411] -> w366
              tunnel: w365 -> [w372 _]
              tunnel: [_ w402] -> w364
              tunnel: [_ w404] -> w363
              tunnel: w362 -> [_ w401]
              tunnel: w361 -> [_ w400]
              frame #0 {
                n125 = stacked-sequence {
                  tunnel: w372 -> [w376]
                  tunnel: w371 -> [w375]
                  tunnel: [w374] -> w369
                  tunnel: [w373] -> w370
                  frame #0 {
                    w388 = cluster{"S/N":string, "USB Search?":bool} {"S/N"="", "USB Search?"=TRUE}  # USB settings
                    w384 = u16 2 items=["RS232", "TCP/IP", "USB"] ("Interface")
                    w383 = cluster{"Portnumber":i32, "Baudrate":u16} {"Portnumber"=0, "Baudrate"=5}  # RS232 settings
                    w382 = T3 {"Host address/name"="", "Port"=50000, "Board"=0, "TCP/IP Search?"=TRUE}  # TCP/IP settings
                    # "TRUE: We want to\nmove the axis to its middle\nposition"
                    # "System number is one"
                    n126 = call "E727_Configuration_Setup.vi"("System no."=w375, "USB settings"=w388, "Are stages connected?"=bool[] [TRUE, TRUE, FALSE], "Change servo status to ON?"=TRUE ("Use dialog to define\nconnected stages?"), "Perform autozero?"=FALSE ("Use dialog to define\nconnected stages?"), "error in"=w376, "Interface"=w384, "RS232 settings"=w383, "TCP/IP settings"=w382, "Stop wave generator\noutput (if any)"=TRUE ("All axes?"), "Move to middle?"=FALSE) -> ("All conn. axes"=w373:string[], "error out"=w378:errorcluster)  [unwired: 3 in, 4 out]
                    n127 = call "POS?.vi"("System no."=w375, "Axes to query"=w373, "All axes?"=TRUE, "error in"=w378) -> ("Position"=→"Position 2":dbl[], "error out"=w374:errorcluster)  [unwired: 1 in, 13 out]
                  }
                }
              }
              frame #1 {
                n128 = for {
                  N: "Number of Steps Left" -> [w414]
                  tunnel: w413 -> [w432]
                  tunnel: [w426] -> w399 mode=indexing
                  tunnel: [w434] -> w411
                  tunnel: w410 -> [w433]
                  tunnel: w409 -> [w431]
                  tunnel: [w430] -> w412
                  tunnel: [w422] -> w403
                  tunnel: [w421] -> w405
                  tunnel: w401 -> [w417]
                  tunnel: w400 -> [w416]
                  stop <- "stop 2" stop-if-true
                  n129 = call <userlib>:"CameraShutter.vi"("Shutter Comp Time: Pre Open"=w416, "error in"=w417, "Shutter State"=3) -> ("Camera Handle"=w419:u32, "error out"=w418:errorcluster)  [unwired: 2 in]
                  n130 = Multiply(x="Step Size (microns)", y=-1) -> (x*y=w427:dbl[])
                  n131 = local write "Step Size (microns)"(w427) -> ()
                  n132 = stacked-sequence {
                    seq-local: [w441 _] -> [_ w545]
                    seq-local: [w442 _] -> [_ w547]
                    tunnel: [_ w546] -> w434
                    tunnel: w433 -> [w445 w548]
                    tunnel: w432 -> [w443 _]
                    tunnel: w431 -> [w444 _]
                    tunnel: [_ w545] -> w430
                    tunnel: [w440 _] -> w424
                    tunnel: [_ w540] -> w415
                    tunnel: [w439 _] -> w422
                    tunnel: [w438 _] -> w421
                    tunnel: w419 -> [w437 _]
                    tunnel: w418 -> [w436 _]
                    frame #0 {
                      n133 = while {
                        shift-right: [w471] -> w449
                        shift-left: dbl[][] [] -> [w476]
                        shift-right: [w474] -> w446
                        shift-left: dbl[][] [] -> [w475]
                        shift-right: [w452] -> w440
                        shift-left: dbl[][] [] -> [w455]
                        tunnel: w444 -> [w473]
                        tunnel: w445 -> [w472]
                        tunnel: w443 -> [w467]
                        tunnel: [w466] -> w442
                        tunnel: [w465] -> w441
                        tunnel: [w462] -> w439
                        tunnel: [w461] -> w438
                        tunnel: w437 -> [w460]
                        tunnel: w436 -> [w459]
                        i -> [w468]
                        stop <- w470 stop-if-true
                        n134 = Increment(x=w468) -> (x+1=w464:i32)
                        n135 = stacked-sequence {
                          tunnel: w473 -> [w494 _]
                          tunnel: [w487 _] -> w466
                          tunnel: w472 -> [w485 _]
                          tunnel: w464 -> [_ _]
                          tunnel: [w480 _] -> w458
                          tunnel: w467 -> [w479 _]
                          tunnel: [w479 _] -> w465
                          tunnel: [_ w499] -> w456
                          tunnel: [_ w498] -> w462
                          tunnel: [_ w497] -> w461
                          tunnel: w460 -> [_ w496]
                          tunnel: w459 -> [_ w495]
                          frame #0 {
                            # "Use first\naxis only."
                            # "Wait until move\nhas stopped or\nstop is pressed"
                            # "Move first axis 0.01 mm\nrelative to its current\nposition."
                            n136 = local read "Step Size (microns)"() -> (w478:dbl[])
                            n137 = Index Array(array=w485, index=0) -> (element=w488:string)
                            n138 = Build Array(w488) -> (w484:string[])
                            n139 = call "MVR.vi"("System no."=w479, "Axes to move"=w484, "Position values"=w478, "error in"=w494) -> ("error out"=w492:errorcluster)  [unwired: 1 in, 14 out]
                            n140 = call "General wait for movement to stop.vi"("System no."=w479, "Axes to wait for"=w484, "error in"=w492) -> ("error out"=w486:errorcluster)  [unwired: 5 in, 11 out]
                            n141 = call "POS?.vi"("System no."=w479, "Axes to query"=w484, "All axes?"=TRUE, "error in"=w486) -> ("Position"=w483:dbl[], "error out"=w491:errorcluster)  [unwired: 1 in, 13 out]
                            "Position" <- w483
                            n142 = Split 1D Array(array=w483, index=1) -> (first subarray=w481:dbl[])  [unwired: 1 out]
                            n143 = call "ERR?.vi"("System no."=w479, "error in"=w491) -> ("error out"=w490:errorcluster)  [unwired: 17 out]
                            n144 = Add Array Elements(numeric array=w481) -> (sum=w480:dbl)
                            n145 = call "GCSTranslateError.vi"("error in"=w490) -> ("error out"=w487:errorcluster)  [unwired: 18 out]
                          }
                          frame #1 {
                            n146 = global read "GlobalFramesToStr.vi" "Frames to Store"() -> (w507:u32)
                            n147 = call "ExSubCreateFile.vi"("error in (no error)"=w495, "Pulser Handle"=u32 0, "Camera Handle"=w496) -> ("error out"=w509:errorcluster, "Handles Out"=w505:T4)  [unwired: 1 in]
                            n148 = Unbundle(w505) -> ("File Handle"=w500:u32, "Image Handle"=w503:u32)  [unwired: 3 out]
                            n149 = call <userlib>:"CameraStart.vi"("error in"=w509) -> ("error out"=w504:errorcluster, "Camera Handle"=w502:u32)  [unwired: 1 in]
                            n150 = for {
                              N: w507 -> [_]
                              tunnel: w504 -> [w514]
                              tunnel: [w513] -> w506
                              tunnel: w500 -> [w512]
                              tunnel: w503 -> [w511]
                              tunnel: [w510] -> w499 mode=indexing
                              n151 = while {
                                tunnel: [w521] -> w513
                                tunnel: w514 -> [w519]
                                tunnel: w512 -> [w518]
                                tunnel: w511 -> [w517]
                                tunnel: [w516] -> w510
                                stop <- w522 stop-if-true
                                n152 = call <userlib>:"CameraCheckData.vi"("error in"=w519) -> ("Camera Handle"=w524:u32, "Number Of Frames Available"=w526:i32, "error out"=w523:errorcluster)  [unwired: 1 in]
                                n153 = Wait Until Next ms Multiple(millisecond multiple=u32 50) -> ()  [unwired: 1 out]
                                n154 = Greater Than 0?(x=w526) -> (x > 0?=w525:bool)
                                n155 = case shown="True" w525 {
                                selector: w525 -> [w527 w537]
                                tunnel: w524 -> [_ w539]
                                tunnel: w523 -> [w528 w538]
                                tunnel: [w527 w537] -> w522
                                tunnel: [w528 w532] -> w521
                                tunnel: w518 -> [_ w531]
                                tunnel: w517 -> [_ w530]
                                tunnel: [_ w529] -> w516
                                frame False {
                                }
                                frame True {
                                w533 = 1
                                n156 = call <userlib>:"CameraGetData.vi"("error in"=w538, "Image/Data Handle"=w530, "Camera Handle"=w539) -> ("error out"=w536:errorcluster, "Image/Data Handle"=w534:u32)  [unwired: 1 out]
                                n157 = call <userlib>:"FileSaveData.vi"("error in"=w536, "Image Handle"=w534, "File Handle"=w531) -> ("error out"=w535:errorcluster)  [unwired: 1 out]
                                n158 = call <userlib>:"ImageGetLineF32.vi"("error in"=w535, "Z Position"=w533, "Y Position"=w533, "Data Handle"=w534) -> ("error out"=w532:errorcluster, "Array F32"=w529:sgl[])  [unwired: 1 out]
                                }
                                }
                              }
                              n159 = Wait Until Next ms Multiple(millisecond multiple=u32 50) -> ()  [unwired: 1 out]
                            }
                            n160 = call <userlib>:"CameraStop.vi"("error in"=w506, "Camera Handle"=w502) -> ("error out"=w508:errorcluster, "Camera Handle"=w497:u32)
                            n161 = call "ExSubCloseFileImage.vi"("error in (no error)"=w508, "Handles In"=w505) -> ("error out"=w498:errorcluster)
                          }
                        }
                        n162 = Greater Or Equal?(x=w464, y="Number of Steps Down") -> (x >= y?=w470:bool)
                        n163 = Insert Into Array(array=w455, new element=w456) -> (w453:dbl[][])  [unwired: 2 in]
                        n164 = Add Array Elements(numeric array=w456) -> (sum=w457:sgl)
                        n165 = Build Array(w457) -> (w477:sgl[])
                        n166 = Build Array(w458, w457) -> (w454:dbl[])
                        n167 = Build Array(w458) -> (w469:dbl[])
                        n168 = Build Array (concatenate)(w453, w454) -> (w452:dbl[][])
                        n169 = Build Array (concatenate)(w476, w469) -> (w471:dbl[][])
                        n170 = Build Array (concatenate)(w475, w477) -> (w474:dbl[][])
                      }
                      n171 = call <vilib>:"Plot Helper.vi"("y matrix"=w446, "x matrix"=w449) -> ("2D Plotmatrix Class Obj Array out"=→"XY Plot Matrix":refnum<class "XY Plot Matrix Datatype.lvclass">[])  [unwired: 2 in, 7 out]
                    }
                    frame #1 {
                      # "Use first\naxis only."
                      # "Wait until move\nhas stopped or\nstop is pressed"
                      # "Move first axis 0.01 mm\nrelative to its current\nposition."
                      n172 = local read "Step Size (microns)"() -> (w542:dbl[])
                      n173 = Index Array(array=w548, index=1) -> (element=w553:string)
                      n174 = Build Array(w553) -> (w551:string[])
                      n175 = Absolute Value(x=w542) -> (abs(x)=w541:dbl[])
                      n176 = call "MVR.vi"("System no."=w545, "Axes to move"=w551, "Position values"=w541, "error in"=w547) -> ("error out"=w557:errorcluster)  [unwired: 1 in, 14 out]
                      n177 = call "General wait for movement to stop.vi"("System no."=w545, "Axes to wait for"=w551, "error in"=w557) -> ("error out"=w552:errorcluster)  [unwired: 5 in, 11 out]
                      n178 = call "POS?.vi"("System no."=w545, "Axes to query"=w551, "All axes?"=TRUE, "error in"=w552) -> ("Position"=w550:dbl[], "error out"=w556:errorcluster)  [unwired: 1 in, 13 out]
                      "Position 3" <- w550
                      n179 = Split 1D Array(array=w550, index=1) -> (second subarray=w543:dbl[])  [unwired: 1 out]
                      n180 = call "ERR?.vi"("System no."=w545, "error in"=w556) -> ("error out"=w555:errorcluster)  [unwired: 17 out]
                      n181 = call "GCSTranslateError.vi"("error in"=w555) -> ("error out"=w546:errorcluster)  [unwired: 18 out]
                      n182 = Split 1D Array(array=w543, index=1) -> (first subarray=w540:dbl[])  [unwired: 1 out]
                    }
                  }
                  n183 = Build Array (concatenate)(w424, w415) -> (w423:dbl[][])
                  n184 = Array To Spreadsheet String(array=w423, 3:"%f" ("format string")) -> (spreadsheet string=w426:string)  [unwired: 1 in]
                  "Line Number" <- w414
                }
                n185 = local read "Number of Steps Left"() -> (w390:dbl)
                n186 = call "File Dialog3"("start path"=path "C:/Users/Raman Lab/Desktop/Molly") -> ("selected path"=w406:path)  [unwired: 11 in, 3 out]
                n187 = local read "Exposure 2"() -> (w393:dbl)
                n188 = call <userlib>:"CameraShutter.vi"("Camera Handle"=w405, "error in"=w403) -> ("Camera Handle"=w404:u32, "error out"=w402:errorcluster)  [unwired: 3 in]
                n189 = local read "Number of Steps Down"() -> (w398:dbl)
                n190 = Number To Decimal String(number=w390) -> (decimal integer string=w389:string)  [unwired: 1 in]
                n191 = Number To Fractional String(number=w398) -> (F-format string=w397:string)  [unwired: 3 in]
                n192 = Number To Decimal String(number=w393) -> (decimal integer string=w394:string)  [unwired: 1 in]
                n193 = Concatenate Strings(w397, "\r\n", w389, "\r\n", w394, "\r\n", w399) -> (w408:string)
                n194 = Write to Text File(file (use dialog)=w406, text=w408) -> ()  [unwired: 2 in, 3 out]
              }
            }
          }
        }
      }
      frame "RF Single Frequency" {
        n195 = case shown="True" "OK Button 4" {
          tunnel: w564 -> [w566 w591]
          tunnel: w562 -> [_ w594]
          tunnel: [w566 w593] -> w561
          tunnel: [w565 w592] -> w560
          tunnel: w563 -> [w565 w590]
          frame False {
          }
          frame True {
            w569 = 1
            n196 = local read "Points"() -> (w586:i32)
            n197 = Initialize Array(0.0, w586, 1.0) -> (w584:dbl[][])
            n198 = for {
              N: "number of scans" -> [_]
              tunnel: w594 -> [w622]
              shift-right: [w621] -> w593
              shift-left: w591 -> [w619]
              shift-right: [w620] -> w592
              shift-left: w590 -> [w618]
              shift-right: [w598] -> _
              shift-left: w584 -> [w601]
              tunnel: [w595] -> w582 mode=indexing
              i -> [w604]
              n199 = call <userlib>:"CameraShutter.vi"("Camera Handle"=w619, "error in"=w618, "Shutter State"=3) -> ("Camera Handle"=w608:u32, "error out"=w609:errorcluster)  [unwired: 2 in]
              n200 = for {
                N: "Points" -> [_]
                shift-right: [w627] -> _
                shift-left: "Frequency" -> [w640]
                tunnel: w622 -> [w643]
                tunnel: [w642] -> w614
                tunnel: [w641] -> w613
                shift-right: [w636] -> _
                shift-left: dbl[][] [] -> [w637]
                tunnel: w609 -> [w639]
                tunnel: w608 -> [w638]
                shift-right: [w629] -> _
                shift-left: dbl[][] [] -> [w633]
                shift-right: [w630] -> w600
                shift-left: dbl[][] [] -> [w632]
                tunnel: [w629] -> w599
                shift-right: [w624] -> w596
                shift-left: dbl[][] [] -> [w625]
                i -> [w623]
                n201 = stacked-sequence {
                  tunnel: w643 -> [w646 _]
                  tunnel: w640 -> [w645 _]
                  tunnel: [_ w655] -> w642
                  tunnel: [_ w656] -> w641
                  tunnel: [w644 _] -> w627
                  tunnel: [_ w654] -> w631
                  tunnel: w639 -> [_ w653]
                  tunnel: w638 -> [_ w652]
                  tunnel: w623 -> [w644 _]
                  frame #0 {
                    n202 = Number To Fractional String(use system decimal point (T)=FALSE, number=w645, precision (6)=7) -> (F-format string=w650:string)  [unwired: 1 in]
                    n203 = Concatenate Strings("f", w650) -> (w651:string)
                    n204 = call "SerialCharWr.vi"("VISA resource name"=w646, "write buffer"=w651) -> ()  [unwired: 6 in, 3 out]
                  }
                  frame #1 {
                    n205 = global read "GlobalFramesToStr.vi" "Frames to Store"() -> (w664:u32)
                    n206 = call "ExSubCreateFile.vi"("error in (no error)"=w653, "Pulser Handle"=u32 0, "Camera Handle"=w652) -> ("error out"=w666:errorcluster, "Handles Out"=w662:T4)  [unwired: 1 in]
                    n207 = Unbundle(w662) -> ("File Handle"=w657:u32, "Image Handle"=w660:u32)  [unwired: 3 out]
                    n208 = call <userlib>:"CameraStart.vi"("error in"=w666) -> ("error out"=w661:errorcluster, "Camera Handle"=w659:u32)  [unwired: 1 in]
                    n209 = for {
                      N: w664 -> [_]
                      tunnel: w661 -> [w671]
                      tunnel: [w670] -> w663
                      tunnel: w657 -> [w669]
                      tunnel: w660 -> [w668]
                      tunnel: [w667] -> w654 mode=indexing
                      n210 = while {
                        tunnel: [w678] -> w670
                        tunnel: w671 -> [w676]
                        tunnel: w669 -> [w675]
                        tunnel: w668 -> [w674]
                        tunnel: [w673] -> w667
                        stop <- w679 stop-if-true
                        n211 = call <userlib>:"CameraCheckData.vi"("error in"=w676) -> ("Camera Handle"=w681:u32, "Number Of Frames Available"=w683:i32, "error out"=w680:errorcluster)  [unwired: 1 in]
                        n212 = Wait Until Next ms Multiple(millisecond multiple=u32 50) -> ()  [unwired: 1 out]
                        n213 = Greater Than 0?(x=w683) -> (x > 0?=w682:bool)
                        n214 = case shown="True" w682 {
                          selector: w682 -> [w684 w694]
                          tunnel: w681 -> [_ w696]
                          tunnel: w680 -> [w685 w695]
                          tunnel: [w684 w694] -> w679
                          tunnel: [w685 w689] -> w678
                          tunnel: w675 -> [_ w688]
                          tunnel: w674 -> [_ w687]
                          tunnel: [_ w686] -> w673
                          frame False {
                          }
                          frame True {
                            w690 = 1
                            n215 = call <userlib>:"CameraGetData.vi"("error in"=w695, "Image/Data Handle"=w687, "Camera Handle"=w696) -> ("error out"=w693:errorcluster, "Image/Data Handle"=w691:u32)  [unwired: 1 out]
                            n216 = call <userlib>:"FileSaveData.vi"("error in"=w693, "Image Handle"=w691, "File Handle"=w688) -> ("error out"=w692:errorcluster)  [unwired: 1 out]
                            n217 = call <userlib>:"ImageGetLineF32.vi"("error in"=w692, "Z Position"=w690, "Y Position"=w690, "Data Handle"=w691) -> ("error out"=w689:errorcluster, "Array F32"=w686:sgl[])  [unwired: 1 out]
                          }
                        }
                      }
                      n218 = Wait Until Next ms Multiple(millisecond multiple=u32 50) -> ()  [unwired: 1 out]
                    }
                    n219 = call <userlib>:"CameraStop.vi"("error in"=w663, "Camera Handle"=w659) -> ("error out"=w665:errorcluster, "Camera Handle"=w655:u32)
                    n220 = call "ExSubCloseFileImage.vi"("error in (no error)"=w665, "Handles In"=w662) -> ("error out"=w656:errorcluster)
                  }
                }
                n221 = Add Array Elements(numeric array=w631) -> (sum=w628:sgl)
                n222 = Insert Into Array(array=w637, new element=w631) -> (w636:dbl[][])  [unwired: 2 in]
                n223 = Build Array(w628) -> (w634:sgl[])
                n224 = Build Array(w627) -> (w635:i32[])
                n225 = Build Array(w628, w627) -> (w626:sgl[])
                n226 = Build Array (concatenate)(w632, w634) -> (w630:dbl[][])
                n227 = Build Array (concatenate)(w633, w635) -> (w629:dbl[][])
                n228 = Build Array (concatenate)(w625, w626) -> (w624:dbl[][])
                "Point #" <- w623
              }
              n229 = Add(x=1, y=w604) -> (x+y=→"Scan #":i32)
              n230 = Add(x=w601, y=w600) -> (x+y=w598:dbl[][])
              "history 2" <- w598
              n231 = call <userlib>:"CameraShutter.vi"("Camera Handle"=w614, "error in"=w613, "Shutter State"=2) -> ("Camera Handle"=w621:u32, "error out"=w620:errorcluster)  [unwired: 2 in]
              n232 = Array To Spreadsheet String(array=w596, 3:"%f" ("format string")) -> (spreadsheet string=w595:string)  [unwired: 1 in]
              n233 = call <vilib>:"Plot Helper.vi"("y matrix"=w598, "x matrix"=w599) -> ("2D Plotmatrix Class Obj Array out"=→"XY Plot Matrix 2":refnum<class "XY Plot Matrix Datatype.lvclass">[])  [unwired: 2 in, 7 out]
            }
            n234 = local read "Frequency"() -> (w579:dbl)
            n235 = local read "number of scans"() -> (w570:i32)
            n236 = local read "Points"() -> (w580:i32)
            n237 = call "File Dialog2"("start path"=path "C:/Users/Raman Lab/Desktop/Molly") -> ("selected path"=w583:path)  [unwired: 11 in, 3 out]
            n238 = Add(x=w579, y=w580) -> (x+y=w568:dbl)
            n239 = Subtract(x=w568, y=w569) -> (x-y=w567:dbl)
            n240 = Number To Fractional String(number=w569) -> (F-format string=w572:string)  [unwired: 3 in]
            n241 = Number To Decimal String(number=w570) -> (decimal integer string=w571:string)  [unwired: 1 in]
            n242 = Number To Fractional String(number=w567) -> (F-format string=w577:string)  [unwired: 3 in]
            n243 = Number To Fractional String(number=w579) -> (F-format string=w578:string)  [unwired: 3 in]
            n244 = Concatenate Strings(w578, "\r\n", w577, "\r\n", w572, "\r\n", w571, "\r\n", w582) -> (w581:string)
            n245 = Write to Text File(file (use dialog)=w583, text=w581) -> ()  [unwired: 2 in, 3 out]
          }
        }
      }
      frame "Stage Control" {
        n246 = case shown="True" "?" {
          tunnel: w697 -> [_ w739]
          tunnel: w698 -> [_ w738]
          frame False {
          }
          frame True {
            n247 = stacked-sequence {
              seq-local: [w741 _] -> [_ w761]
              seq-local: [w740 _] -> [_ w760]
              tunnel: w738 -> [w742 _]
              tunnel: w739 -> [w743 _]
              frame #0 {
                n248 = stacked-sequence {
                  tunnel: w743 -> [w747]
                  tunnel: w742 -> [w746]
                  tunnel: [w745] -> w740
                  tunnel: [w744] -> w741
                  frame #0 {
                    w759 = cluster{"S/N":string, "USB Search?":bool} {"S/N"="", "USB Search?"=TRUE}  # USB settings
                    w755 = u16 2 items=["RS232", "TCP/IP", "USB"] ("Interface")
                    w754 = cluster{"Portnumber":i32, "Baudrate":u16} {"Portnumber"=0, "Baudrate"=5}  # RS232 settings
                    w753 = T3 {"Host address/name"="", "Port"=50000, "Board"=0, "TCP/IP Search?"=TRUE}  # TCP/IP settings
                    # "TRUE: We want to\nmove the axis to its middle\nposition"
                    # "System number is one"
                    n249 = call "E727_Configuration_Setup.vi"("System no."=w746, "USB settings"=w759, "Are stages connected?"=bool[] [TRUE, TRUE, FALSE], "Change servo status to ON?"=TRUE ("Use dialog to define\nconnected stages?"), "Perform autozero?"=FALSE ("Use dialog to define\nconnected stages?"), "error in"=w747, "Interface"=w755, "RS232 settings"=w754, "TCP/IP settings"=w753, "Stop wave generator\noutput (if any)"=TRUE ("All axes?"), "Move to middle?"=FALSE) -> ("All conn. axes"=w744:string[], "error out"=w749:errorcluster)  [unwired: 3 in, 4 out]
                    n250 = call "POS?.vi"("System no."=w746, "Axes to query"=w744, "All axes?"=TRUE, "error in"=w749) -> ("Position"=→"Position 4":dbl[], "error out"=w745:errorcluster)  [unwired: 1 in, 13 out]
                  }
                }
              }
              frame #1 {
                n251 = stacked-sequence {
                  tunnel: w761 -> [w764]
                  tunnel: w760 -> [w763]
                  frame #0 {
                    w762 = 1
                    # "Use first\naxis only."
                    # "Wait until move\nhas stopped or\nstop is pressed"
                    # "Move first axis 0.01 mm\nrelative to its current\nposition."
                    n252 = local read "Step Size (microns) Y"() -> (w765:dbl[])
                    n253 = Index Array(array=w764, index=0) -> (element=w769:string)
                    n254 = Build Array(w769) -> (w767:string[])
                    n255 = call "MVR.vi"("System no."=w762, "Axes to move"=w767, "Position values"=w765, "error in"=w763) -> ("error out"=w773:errorcluster)  [unwired: 1 in, 14 out]
                    n256 = call "General wait for movement to stop.vi"("System no."=w762, "Axes to wait for"=w767, "error in"=w773) -> ("error out"=w768:errorcluster)  [unwired: 5 in, 11 out]
                    n257 = call "POS?.vi"("System no."=w762, "Axes to query"=w767, "All axes?"=TRUE, "error in"=w768) -> ("Position"=→"Position 5":dbl[], "error out"=w772:errorcluster)  [unwired: 1 in, 13 out]
                    n258 = call "ERR?.vi"("System no."=w762, "error in"=w772) -> ("error out"=w771:errorcluster)  [unwired: 17 out]
                    n259 = call "GCSTranslateError.vi"("error in"=w771) -> ()  [unwired: 19 out]
                  }
                }
              }
            }
          }
        }
        n260 = case shown="True" "?" {
          tunnel: w697 -> [_ w702]
          tunnel: w698 -> [_ w701]
          frame False {
          }
          frame True {
            n261 = stacked-sequence {
              seq-local: [w704 _] -> [_ w724]
              seq-local: [w703 _] -> [_ w723]
              tunnel: w701 -> [w705 _]
              tunnel: w702 -> [w706 _]
              frame #0 {
                n262 = stacked-sequence {
                  tunnel: w706 -> [w710]
                  tunnel: w705 -> [w709]
                  tunnel: [w708] -> w703
                  tunnel: [w707] -> w704
                  frame #0 {
                    w722 = cluster{"S/N":string, "USB Search?":bool} {"S/N"="", "USB Search?"=TRUE}  # USB settings
                    w718 = u16 2 items=["RS232", "TCP/IP", "USB"] ("Interface")
                    w717 = cluster{"Portnumber":i32, "Baudrate":u16} {"Portnumber"=0, "Baudrate"=5}  # RS232 settings
                    w716 = T3 {"Host address/name"="", "Port"=50000, "Board"=0, "TCP/IP Search?"=TRUE}  # TCP/IP settings
                    # "TRUE: We want to\nmove the axis to its middle\nposition"
                    # "System number is one"
                    n263 = call "E727_Configuration_Setup.vi"("System no."=w709, "USB settings"=w722, "Are stages connected?"=bool[] [TRUE, TRUE, FALSE], "Change servo status to ON?"=TRUE ("Use dialog to define\nconnected stages?"), "Perform autozero?"=FALSE ("Use dialog to define\nconnected stages?"), "error in"=w710, "Interface"=w718, "RS232 settings"=w717, "TCP/IP settings"=w716, "Stop wave generator\noutput (if any)"=TRUE ("All axes?"), "Move to middle?"=FALSE) -> ("All conn. axes"=w707:string[], "error out"=w712:errorcluster)  [unwired: 3 in, 4 out]
                    n264 = call "POS?.vi"("System no."=w709, "Axes to query"=w707, "All axes?"=TRUE, "error in"=w712) -> ("Position"=→"Position 7":dbl[], "error out"=w708:errorcluster)  [unwired: 1 in, 13 out]
                  }
                }
              }
              frame #1 {
                n265 = stacked-sequence {
                  tunnel: w724 -> [w727]
                  tunnel: w723 -> [w726]
                  frame #0 {
                    w725 = 1
                    # "Use first\naxis only."
                    # "Wait until move\nhas stopped or\nstop is pressed"
                    # "Move first axis 0.01 mm\nrelative to its current\nposition."
                    n266 = local read "Step Size (microns) X"() -> (w728:dbl[])
                    n267 = Index Array(array=w727, index=1) -> (element=w732:string)
                    n268 = Build Array(w732) -> (w730:string[])
                    n269 = call "MVR.vi"("System no."=w725, "Axes to move"=w730, "Position values"=w728, "error in"=w726) -> ("error out"=w736:errorcluster)  [unwired: 1 in, 14 out]
                    n270 = call "General wait for movement to stop.vi"("System no."=w725, "Axes to wait for"=w730, "error in"=w736) -> ("error out"=w731:errorcluster)  [unwired: 5 in, 11 out]
                    n271 = call "POS?.vi"("System no."=w725, "Axes to query"=w730, "All axes?"=TRUE, "error in"=w731) -> ("Position"=→"Position 8":dbl[], "error out"=w735:errorcluster)  [unwired: 1 in, 13 out]
                    n272 = call "ERR?.vi"("System no."=w725, "error in"=w735) -> ("error out"=w734:errorcluster)  [unwired: 17 out]
                    n273 = call "GCSTranslateError.vi"("error in"=w734) -> ()  [unwired: 19 out]
                  }
                }
              }
            }
          }
        }
      }
    }
    n274 = global read "GlobalCamOpen.vi" "Camera Opened"() -> (w25:u32)
    n275 = Not(x="Release Camera") -> (.not. x?=w17:bool)
    n276 = Greater Than 0?(x=w25) -> (x > 0?=w24:bool)
    n277 = And(x=w17, y=w24) -> (x .and. y?=→"Camera Opened":bool)
    n278 = Wait Until Next ms Multiple(millisecond multiple=5) -> ()  [unwired: 1 out]
  }
  n279 = call <userlib>:"CameraClose.vi"("error in"=w8, "Camera Handle"=w5) -> ("error out"=w7:errorcluster)
  n280 = call "Close connection if open.vi"("System no."=w1) -> ("error out"=→"error out 2":errorcluster)  [unwired: 2 in, 16 out]
  n281 = call <userlib>:"UninitToolkit.vi"("error in"=w7) -> ("error out"=→"error out":errorcluster)
